vi "testparallel.vi"   [LabVIEW 2017]
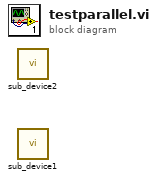
[diagram p0: block diagram]
diagram:
  n1 = call "sub_device2.vi"() -> ()  [unwired: 12 in]
  n2 = call "sub_device1.vi"() -> ()  [unwired: 12 in]
